vi "ChannelTypetoClass.vi"(11 "channel name":string) -> (3 "string":string)   [LabVIEW 2013, in "_Group.lvclass"]
uses:
  _Group.lvclass
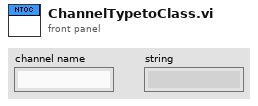
[diagram p1: front panel]
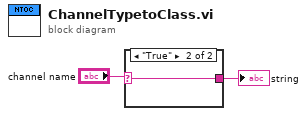
[diagram p0: block diagram]
diagram:
  n1 = case shown="\"True\"" "channel name" {
    selector: "channel name" -> [_ w3]
    tunnel: [_ w3] -> w2
    frame "False", Default {
    }
    frame "True" {
    }
  }
  "string" <- w2
